vi "GUI_BELLA_HamamatsuSpec.vi"() -> ()   [LabVIEW 2013]
uses:
  Shared/GUI_Template/GUI_master/tcp_new_data_event.ctl
  Shared/GUI_Template/GUI_master/tcp new data cluster.ctl
panel:
  in  "save::1":bool caption="Blank Button"
  in  "trigger::1":bool caption="Blank Button"
  out "XY Graph":cluster{"counts":dbl[], "wavelength":dbl[]}(graph)
  in  "wavelength::1":dbl[](array[numeric]) caption="wavelength"
  in  "counts::1":dbl[](array[numeric]) caption="counts"
  out "tcp data event":T1
  out "error IO 2":errorcluster
  in  "GUIdevice 1":string="BellaHamamatsuSpec"
  in  "insert tag":bool=TRUE
  in  "stop":bool
  # "BELLA HAMAMATSU SPECTROMETER"
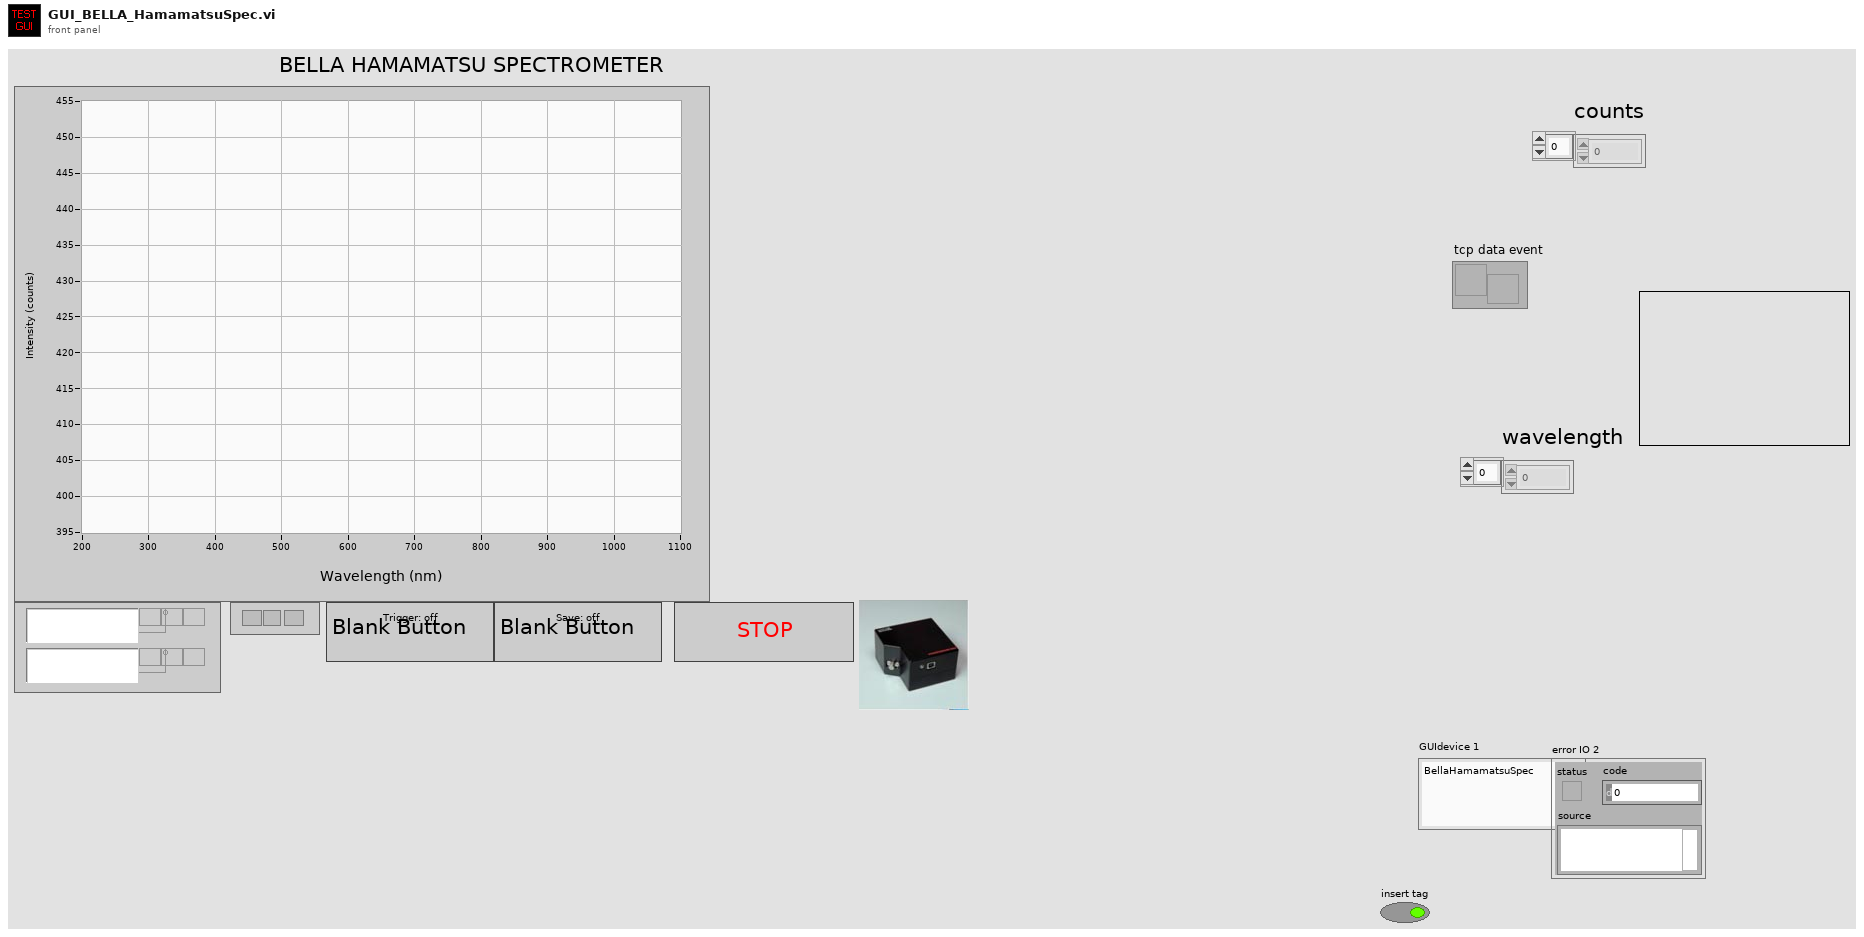
[diagram p1: front panel]
types:
  T1 = typedef "tcp_new_data_event.ctl" = refnum<user-event>
  T2 = typedef "tcp new data cluster.ctl" = cluster{"EventEnum":enum16{"new data", "connection status update"}, "Device name":string}
  T3 = cluster{"wavelength::1":dbl[], "counts::1":dbl[]}
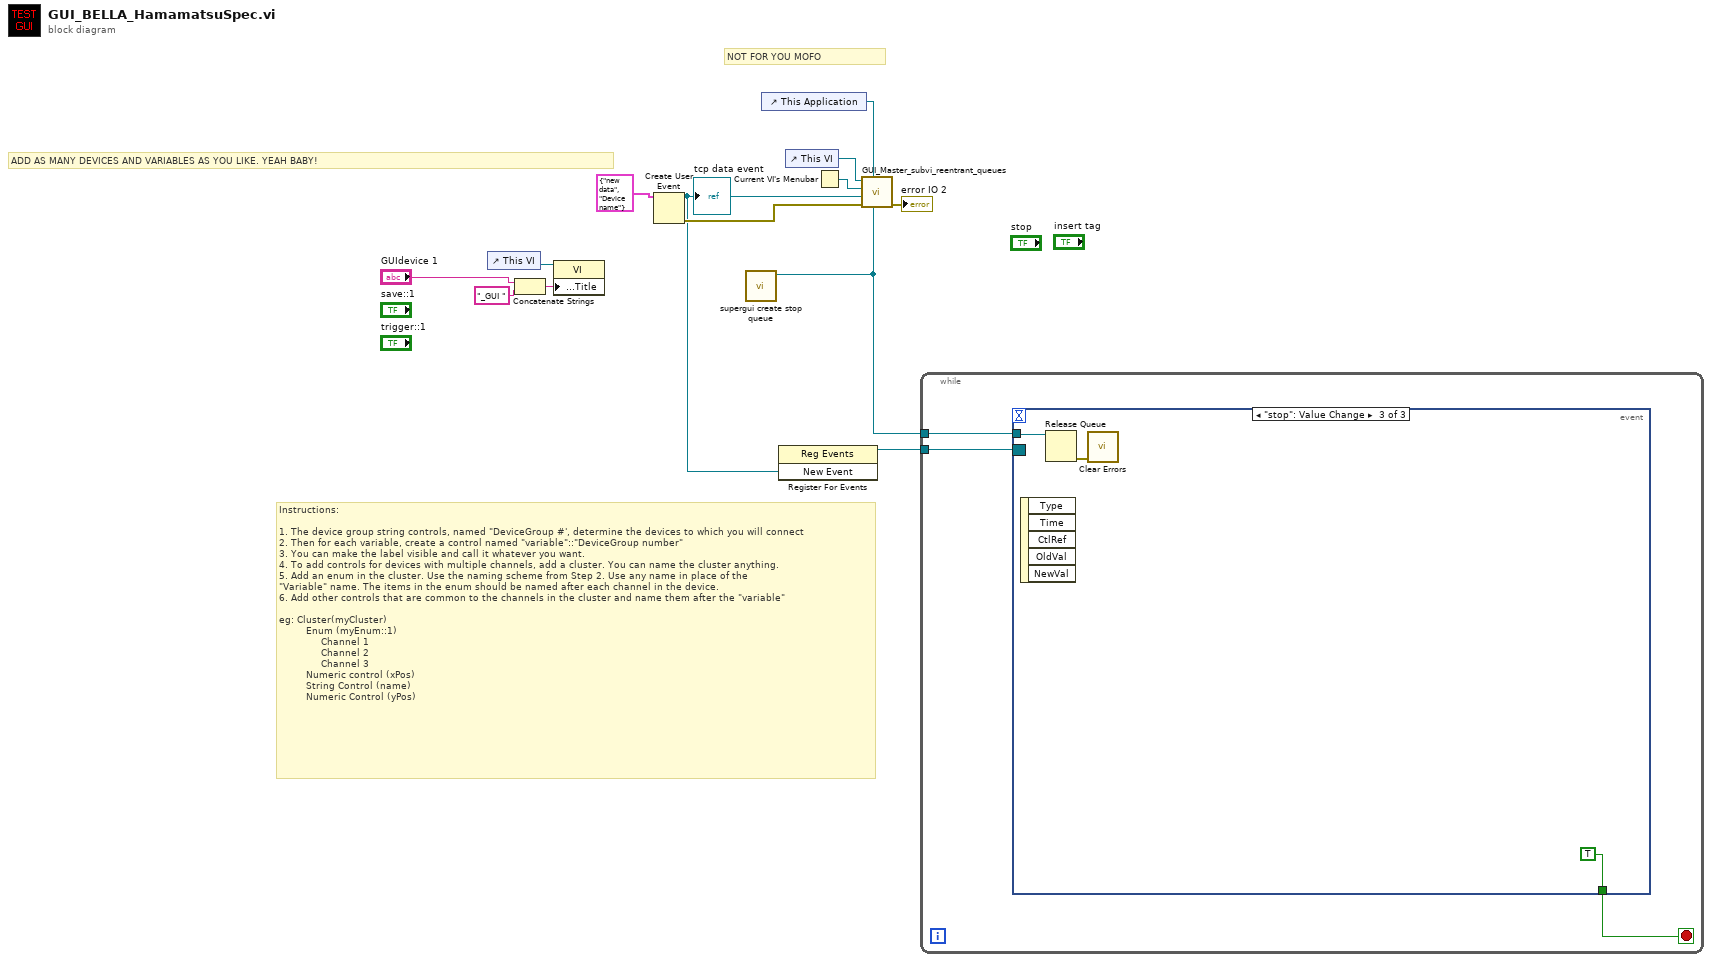
[diagram p0: block diagram]
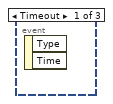
[diagram p2: hidden frame]
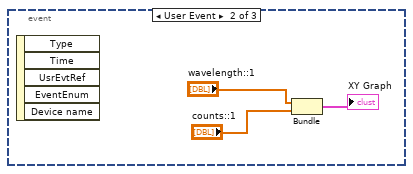
[diagram p3: hidden frame]
diagram:
  # "Instructions:\n\n1. The device group string controls, named \"DeviceGroup #', determine the devices to which you will connect\n2. Then for each variable, create a control named \"variable\"::\"DeviceGroup number\"\n3. You can make the label visible and call it whatever you want.\n4. To add controls for devices with multiple channels, add a cluster. You can name the cluster anything.\n5. Add an enum in the cluster. Use the naming scheme from Step 2. Use any name in place of the \n\"Variable\" name. The items in the enum should be named after each channel in the device. \n6. Add other controls that are common to the channels in the cluster and name them after the \"variable\"\n\neg: Cluster(myCluster)\n         Enum (myEnum::1)\n              Channel 1 \n              Channel 2\n              Channel 3\n         Numeric control (xPos)\n         String Control (name)\n         Numeric Control (yPos)"
  # "ADD AS MANY DEVICES AND VARIABLES AS YOU LIKE. YEAH BABY!"
  # "NOT FOR YOU MOFO"
  n1 = control-ref of="This VI"() -> (w4:refnum<vi>)
  n2 = Concatenate Strings("GUIdevice 1", "_GUI ") -> (w3:string)
  n3 = property class="VI"(reference=w4, "Front Panel.Title"=w3) -> ()  [unwired: 1 in, 2 out]
  n4 = Create User Event(user event datatype=T2 {"EventEnum"=enum."new data", "Device name"="Device name"} ("New Event")) -> (user event=w7:refnum<user-event>, error out=w9:errorcluster)  [unwired: 1 in]
  "tcp data event" <- w7
  n5 = call "supergui create stop queue.vi"() -> ("STOP Queue out"=w5:refnum<queue>)  [unwired: 11 in]
  n6 = control-ref of="This Application"() -> (w8:refnum<vi>)
  n7 = register-events(w7) -> (reference out=w6:refnum<event-registration>)  [unwired: 2 in, 1 out]
  n8 = control-ref of="This VI"() -> (w12:refnum<vi>)
  n9 = Current VI's Menubar() -> (w11:refnum<k9>)
  n10 = call "GUI_Master_subvi_reentrant_queues.vi"("STOP Queue in"=w5, "This Application"=w8, "error in (no error)"=w9, "tcp data event"=w7, "Caller menu reference"=w11, "Caller VI ref"=w12) -> ("error out"=→"error IO 2":errorcluster)  [unwired: 5 in]
  n11 = while {
    tunnel: w6 -> [w15]
    tunnel: w5 -> [w14]
    stop <- w16 stop-if-true
    n12 = event shown="[2] \"stop\": Value Change" {
      selector: w15 -> [_ _ _]
      dyn-events: _ -> [_ _ _]
      timeout: _ -> [_ _ _]
      tunnel: [_ _ TRUE] -> w16
      tunnel: w14 -> [_ _ w21]
      event Timeout {
        n13 = event-data() -> ()  [unwired: 1 in, 2 out]
      }
      event User Event {
        n14 = event-data() -> ()  [unwired: 1 in, 5 out]
        n15 = Bundle("wavelength::1"="wavelength::1", "counts::1"="counts::1") -> (→"XY Graph":T3)  [unwired: 1 in]
      }
      event "stop": Value Change {
        n16 = event-data() -> ()  [unwired: 1 in, 5 out]
        n17 = Release Queue(queue=w21) -> (error out=w20:errorcluster)  [unwired: 2 in, 2 out]
        n18 = call <vilib>:"Clear Errors.vi"("error in (no error)"=w20) -> ()  [unwired: 6 in, 1 out]
      }
    }
  }
